vi "SH_generateShapelets.vi"(5 "MaxLength (in %)":dbl(slide) min=0.0 max=1.0 step=0.05 scale=0.0..1.0, 7 "MinLength (in %)":dbl(slide) min=0.0 max=1.0 step=0.05 scale=0.0..1.0, 8 "error in (no error)":errorcluster, 9 "Progress":refnum<vi>, 10 "Shapelets Queue":refnum<queue>, 11 "ShapeletClass in":refnum<class "Shapelets Search Brute Force.lvclass">) -> (0 "error out":errorcluster, 2 "Total Number of Shapelets":i32, 3 "ShapeletClass out":refnum<class "Shapelets Search Brute Force.lvclass">)   [LabVIEW 2016, in "Shapelets Search (Brute Force).lvlib" / "Shapelets Search Brute Force.lvclass"]
uses:
  Shapelets Search Brute Force.lvclass
  SH_Shapelet.ctl
  Shapelets Search Brute Force.lvclass/Shapelets Search Brute Force.ctl
  Shapelets Search (Brute Force).lvlib
panel:
  # "This VI is a part of BCI Design library, http://www.ru-bci.org \nCopyright © 2020, Sotnikov Peter, All rights reserved. License: CC BY-NC 4.0"
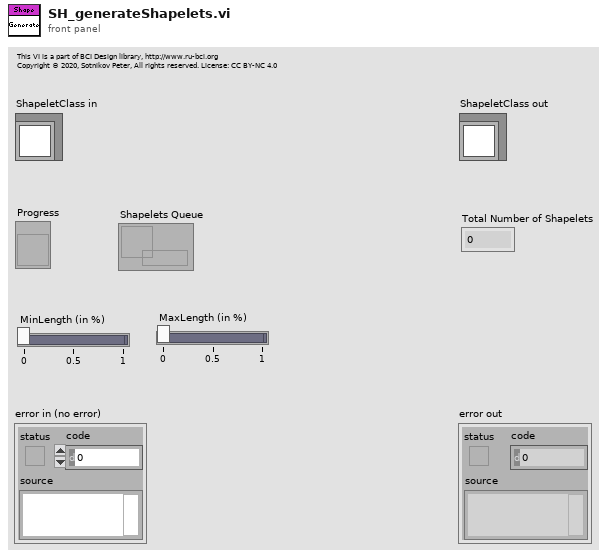
[diagram p1: front panel]
types:
  T1 = typedef "Shapelets Search (Brute Force).lvlib/SH_Shapelet.ctl" = cluster{"TrialIndex":i32, "Shift (in samples)":i32, "Length (in samples)":i32, "Distances":dbl[], "ClassIndecies":i32[], "Fitness":dbl, "Split Point":dbl}
  T2 = cluster{"ClassLabel":string, "FeatureVector":dbl[][]}[]
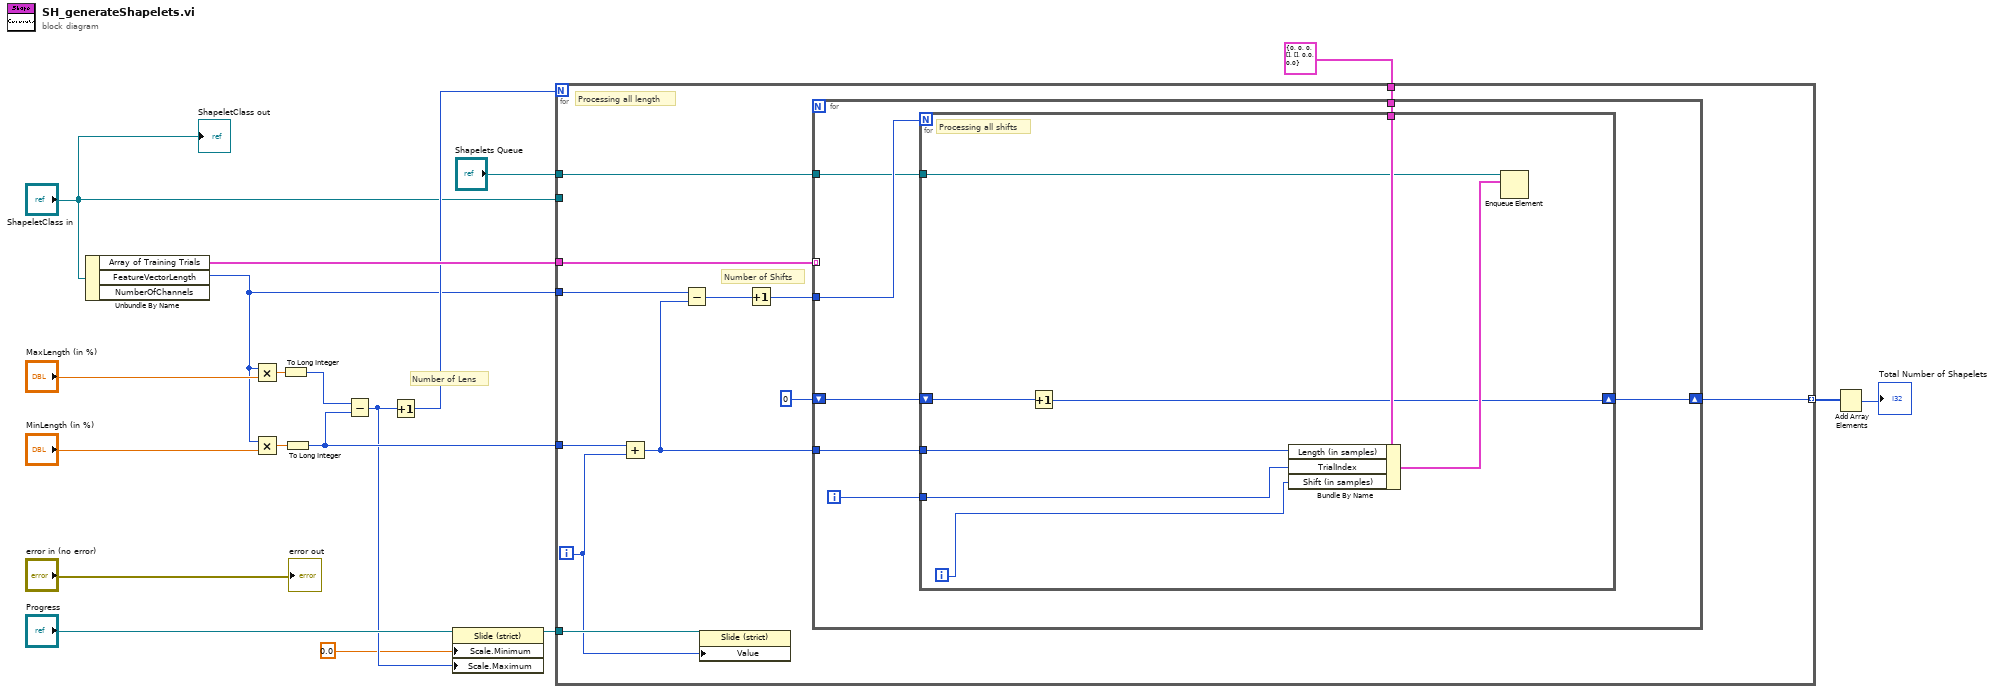
[diagram p0: block diagram]
diagram:
  # "Number of Lens"
  n1 = Unbundle By Name("ShapeletClass in") -> ("Array of Training Trials"=w12:T2, "FeatureVectorLength"=w1:i32)  [unwired: 1 out]
  n2 = Multiply(x=w1, y="MaxLength (in %)") -> (x*y=w15:dbl)
  n3 = Multiply(x=w1, y="MinLength (in %)") -> (x*y=w14:dbl)
  n4 = To Long Integer(number=w15) -> (32bit integer=w13:i32)
  n5 = To Long Integer(number=w14) -> (32bit integer=w11:i32)
  n6 = Subtract(x=w13, y=w11) -> (x-y=w4:i32)
  n7 = Increment(x=w4) -> (x+1=w8:i32)
  n8 = property class="Slide (strict)"(reference="Progress", "Scale.Minimum"=0.0 ("Data Entry Limits:Minimum"), "Scale.Maximum"=w4) -> (reference out=w9:refnum<vi>)  [unwired: 1 in, 1 out]
  n9 = for {
    N: w8 -> [_]
    tunnel: w12 -> [w27]
    tunnel: w11 -> [w31]
    tunnel: w1 -> [w30]
    tunnel: w9 -> [w25]
    tunnel: T1 {"TrialIndex"=0, "Shift (in samples)"=0, "Length (in samples)"=0, "Distances"=[], "ClassIndecies"=[], "Fitness"=0.0, "Split Point"=0.0} ("Shapelet") -> [w23]
    tunnel: "ShapeletClass in" -> [_]
    tunnel: "Shapelets Queue" -> [w22]
    tunnel: [w20] -> w2 mode=indexing
    i -> [w24]
    # "Number of Shifts"
    # "Processing all length"
    n10 = Add(x=w31, y=w24) -> (x+y=w28:i32)
    n11 = Subtract(x=w30, y=w28) -> (x-y=w29:i32)
    n12 = property class="Slide (strict)"(reference=w25, "Value"=w24) -> ()  [unwired: 1 in, 2 out]
    n13 = Increment(x=w29) -> (x+1=w26:i32)
    n14 = for {
      tunnel: w28 -> [w38]
      tunnel: w27 -> [_] mode=indexing
      tunnel: w26 -> [w37]
      tunnel: w23 -> [w35]
      tunnel: w22 -> [w34]
      shift-right: [w32] -> w20
      shift-left: 0 -> [w33]
      i -> [w36]
      n15 = for {
        N: w37 -> [_]
        tunnel: w38 -> [w46]
        tunnel: w36 -> [w45]
        tunnel: w35 -> [w43]
        tunnel: w34 -> [w42]
        shift-right: [w39] -> w32
        shift-left: w33 -> [w40]
        i -> [w44]
        # "Processing all shifts"
        n16 = Increment(x=w40) -> (x+1=w39:i32)
        n17 = Bundle By Name(cluster=w43, "Length (in samples)"=w46, "TrialIndex"=w45, "Shift (in samples)"=w44) -> (w41:T1)
        n18 = Enqueue Element(queue=w42, element=w41) -> ()  [unwired: 2 in, 3 out]
      }
    }
  }
  n19 = Add Array Elements(numeric array=w2) -> (sum=→"Total Number of Shapelets":i32)
  "error out" <- "error in (no error)"
  "ShapeletClass out" <- "ShapeletClass in"
